vi "Do Command.vi"(6 "Actions In":refnum<class "Iteration Actions.lvclass">, 7 "Variables in":refnum<class "Variables.lvclass">, 8 "error in (no error)":errorcluster, 9 "Sequence Time":T1, 10 "VolatusAPI":refnum<class "VolatusAPI.lvclass">, 11 "Transition Command in":refnum<class "Transition Command.lvclass">) -> (0 "error out":errorcluster, 4 "Actions":refnum<class "Iteration Actions.lvclass">, 5 "Variables":refnum<class "Variables.lvclass">)   [LabVIEW 2020, in "VolatusSeq.lvlib" / "Transition Command.lvclass"]
uses:
  Transition Command.lvclass
  Variables/Variables.lvclass
  Volatus/VolatusAPI/VolatusAPI.lvclass
  Iteration Actions/Iteration Actions.lvclass
  Transition Command.lvclass/Transition Command.ctl
  Iteration Actions/Iteration Actions.lvclass/Iteration Actions.ctl
  Sequence Time.ctl
  VolatusSeq.lvlib
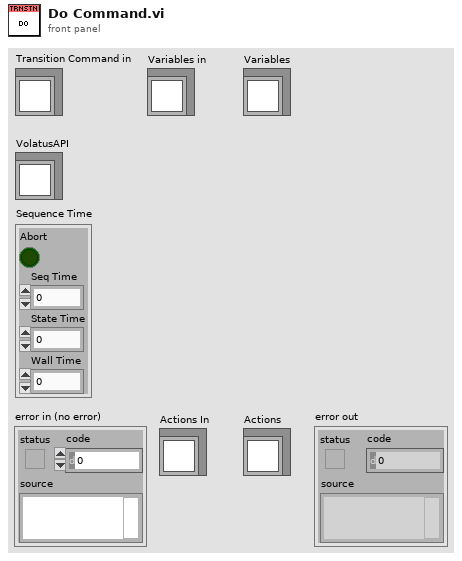
[diagram p1: front panel]
types:
  T1 = typedef "VolatusSeq.lvlib/Sequence Time.ctl" = cluster{"Abort":bool, "Seq Time":dbl, "State Time":dbl, "Wall Time":dbl}
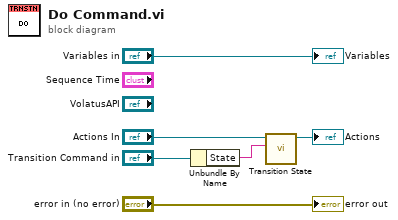
[diagram p0: block diagram]
diagram:
  n1 = Unbundle By Name("Transition Command in") -> ("State"=w3:string)
  n2 = call "Transition State.vi"("Next State"=w3, "Iteration Actions in"="Actions In") -> ("Iteration Actions out"=→"Actions":refnum<class "Iteration Actions.lvclass">)  [unwired: 8 in, 1 out]
  "error out" <- "error in (no error)"
  "Variables" <- "Variables in"
